vi "Messages GUI.vi"(11 "Messages":string) -> ()   [LabVIEW 2021, in "CANOpen Addon System Explorer.lvlib"]
uses:
  CANOpen Addon System Explorer.lvlib
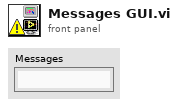
[diagram p1: front panel]
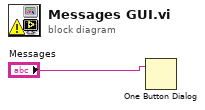
[diagram p0: block diagram]
diagram:
  n1 = One Button Dialog(message="Messages") -> ()  [unwired: 1 in, 1 out]
